vi "digital read.vi"(8 "error in (no error)":errorcluster, 10 "Line":string, 11 "USB-6000 in":refnum<class "USB-6000.lvclass">) -> (0 "error out":errorcluster, 2 "High/Low":bool, 3 "USB-6000 out":refnum<class "USB-6000.lvclass">)   [LabVIEW 2025, in "USB IO.lvlib" / "USB-6000.lvclass"]
uses:
  USB-6000.lvclass
  USB-6000.lvclass/USB-6000.ctl
  <vilib>/DAQmx/read.llb/DAQmx Read (Digital Bool 1Line 1Point).vi
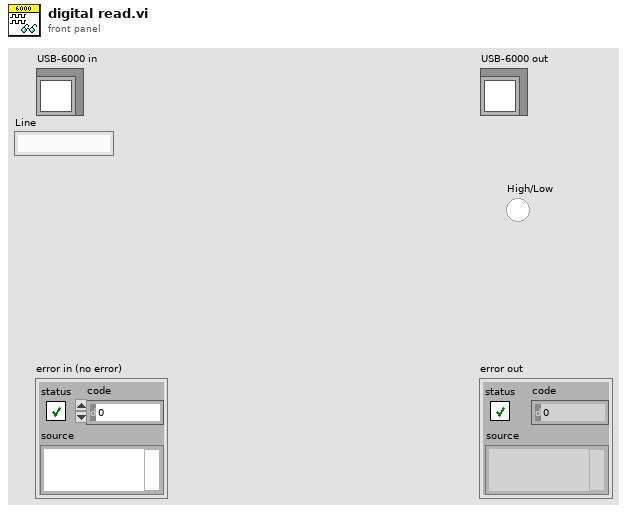
[diagram p1: front panel]
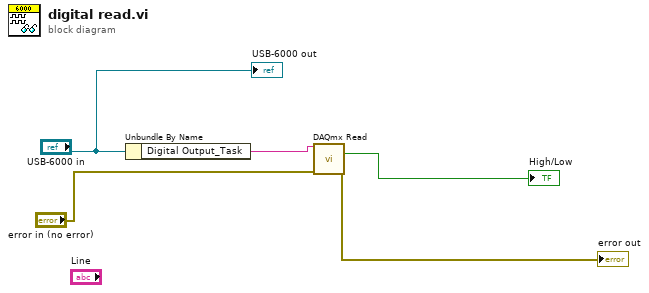
[diagram p0: block diagram]
diagram:
  n1 = Unbundle By Name("USB-6000 in") -> ("Digital Output_Task"=w4:string)
  n2 = call-poly <vilib>:"DAQmx Read.vi"("task/channels in"=w4, "error in"="error in (no error)") -> ("data"=→"High/Low":bool, "error out"=→"error out":errorcluster)  [unwired: 11 in, 1 out]
  "USB-6000 out" <- "USB-6000 in"
